vi "SVXMPL_Build Orbit PLot (spectrum).vi"(0 "real part [EUy/EUx rms]":cluster{"f0":dbl, "df":dbl, "real part":dbl[]} {"real part" format="%.2f"; "df" format="%.2f"; "f0" format="%.2f"}, 2 "imaginary part [EUy/EUx rms]":T1 {"imaginary part" format="%.2f"; "df" format="%.2f"; "f0" format="%.2f"}, 5 "error in (no error)":errorcluster) -> (14 "Nyquist Plot":cluster{"Y":dbl[], "Y":dbl[]}(graph), 19 "error out":errorcluster)   [LabVIEW 2017]
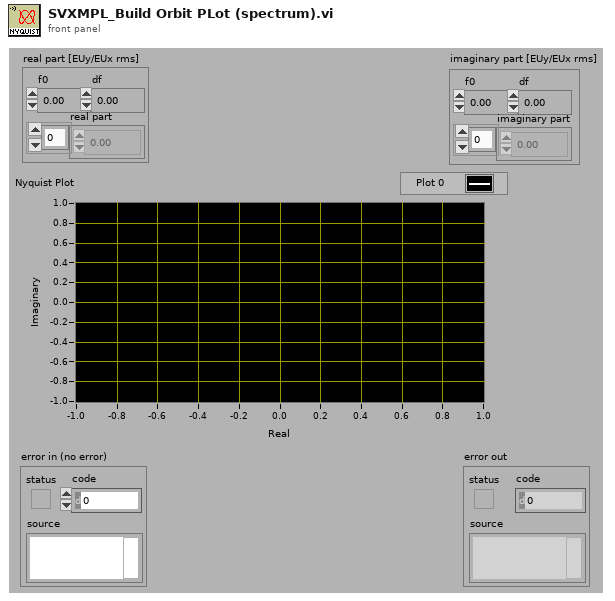
[diagram p1: front panel]
types:
  T1 = cluster{"f0":dbl, "df":dbl, "imaginary part":dbl[]}
  T2 = cluster{"real part":dbl[], "imaginary part":dbl[]}
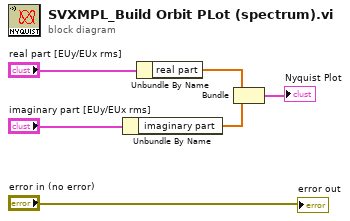
[diagram p0: block diagram]
diagram:
  n1 = Unbundle By Name("imaginary part [EUy/EUx rms]") -> ("imaginary part"=w1:dbl[])
  n2 = Unbundle By Name("real part [EUy/EUx rms]") -> ("real part"=w2:dbl[])
  n3 = Bundle("real part"=w2, "imaginary part"=w1) -> (→"Nyquist Plot":T2)  [unwired: 1 in]
  "error out" <- "error in (no error)"
